vi "Entry.vi"(8 "error in (no error)":errorcluster, 11 "New State":refnum<class "GTH-Up.lvclass">) -> (0 "error out":errorcluster, 3 "State out":refnum<class "GTH-Up.lvclass">)   [LabVIEW 2014, in "Elevator.lvlib" / "EL-Go To Height.lvlib" / "GTH-Up.lvclass"]
doc: "This is an abstract method. Override this method to define the behavior when you enter the state."
uses:
  GTH-Up.lvclass
  Elevator Messages/Set Rate (Percent) Msg/Set Rate (Percent) Msg.lvclass/Set Rate (Percent) Msg.ctl
  <vilib>/ActorFramework/Message Enqueuer/Message Enqueuer.lvclass/Message Enqueuer.ctl
  <vilib>/ActorFramework/Message Enqueuer/Enqueue.vi
  <vilib>/ActorFramework/Message Priority Queue/Priority Enqueue.vi
  EL-Go To Height Class/EL-Go To Height.lvclass
  Elevator Messages/Set Rate (Percent) Msg/Set Rate (Percent) Msg.lvclass
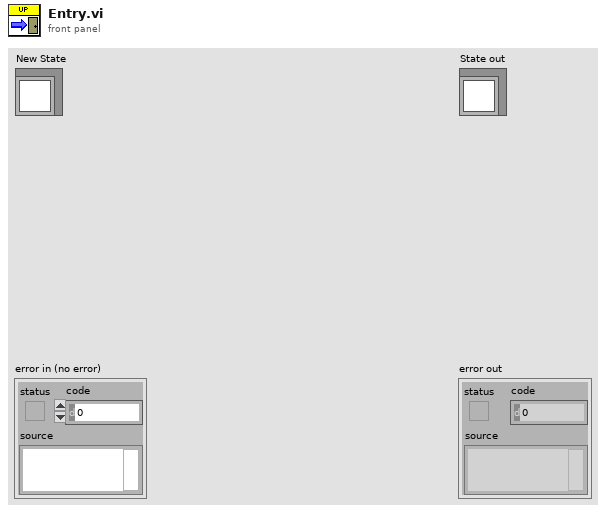
[diagram p1: front panel]
types:
  T1 = typedef "Elevator.lvlib/EL-Go To Height.lvlib/EL-Go To Height.lvclass/Parameters.ctl" = cluster{"Target Height":dbl, "Elevator State Loop (ms)":u32, "Up Rate (Percentage)":dbl, "Down Rate (Percentage)":dbl}
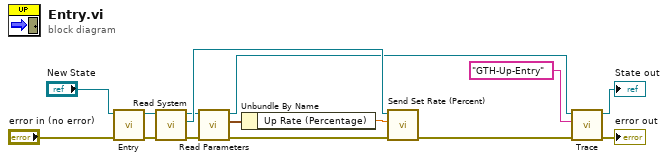
[diagram p0: block diagram]
diagram:
  n1 = call-parent "Entry.vi"("error in (no error)"="error in (no error)", "New State"="New State") -> ("error out"=w5:errorcluster, "State out"=w10:refnum<class "GTH-Up.lvclass">)  [unwired: 8 in]
  n2 = call-dynamic "Read System.vi"("error in (no error)"=w5, "Command in"=w10) -> ("error out"=w4:errorcluster, "Actor Framework:Message Enqueuer"=w9:refnum<class "Message Enqueuer.lvclass">, "Command out"=w8:refnum<class "GTH-Up.lvclass">)  [unwired: 7 in]
  n3 = call-dynamic "Read Parameters.vi"("error in (no error)"=w4, "EL-Go To Height in"=w8) -> ("error out"=w3:errorcluster, "Parameters"=w7:T1, "EL-Go To Height out"=w1:refnum<class "GTH-Up.lvclass">)  [unwired: 7 in]
  n4 = Unbundle By Name(w7) -> ("Up Rate (Percentage)"=w6:dbl)
  n5 = call "Send Set Rate (Percent).vi"("error in (no error)"=w3, "Percent"=w6, "Message Enqueuer"=w9) -> ("error out"=w2:errorcluster)  [unwired: 7 in, 1 out]
  n6 = call-dynamic "Trace.vi"("error in (no error)"=w2, "Command Action"="GTH-Up-Entry", "Command Actor in"=w1) -> ("error out"=→"error out":errorcluster, "Command Actor out"=→"State out":refnum<class "GTH-Up.lvclass">)  [unwired: 7 in]
